vi "Items.vi"(8 "error in (no error)":errorcluster, 11 "MockListImp in":refnum<class "ListImp_RefSpy.lvclass">) -> (0 "error out":errorcluster, 1 "Items":refnum<class>[](array[class]), 3 "MockListImp out":refnum<class "ListImp_RefSpy.lvclass">)   [LabVIEW 2013, in "ListImp_RefSpy.lvclass"]
uses:
  ListImp_RefSpy.lvclass
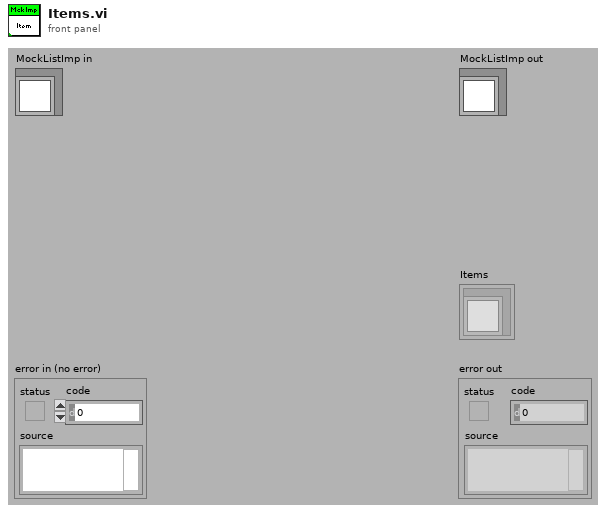
[diagram p1: front panel]
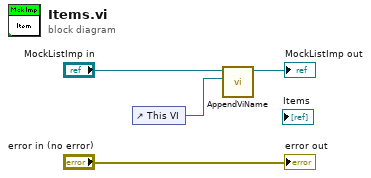
[diagram p0: block diagram]
diagram:
  n1 = control-ref of="This VI"() -> (w1:refnum<vi>)
  n2 = call "AppendViName.vi"("VI Refnum"=w1, "MockListImp in"="MockListImp in") -> ("MockListImp out"=→"MockListImp out":refnum<class "ListImp_RefSpy.lvclass">)  [unwired: 8 in, 1 out]
  "error out" <- "error in (no error)"
